vi "Configure Basic Clock Reference.vi"(5 "AES Termination Status (T: Enable)":bool=TRUE, 6 "BNC Termination Status (T: Enable)":bool=TRUE, 7 "Delay Output From Reference (0 s)":dbl, 8 "error in (no error)":errorcluster, 9 "Enable Clock Lock (T: Enable)":bool=TRUE, 10 "Clock Source (0: crAES)":i32(ring) items=["crAES", "crExt", "crInt", "crNTSC", "crSECAM", "crPAL"], 11 "VISA resource name":refnum<visa-resource-name>) -> (0 "error out":errorcluster, 3 "VISA resource name out":refnum<visa-resource-name>)   [LabVIEW 2014, in "Stanford Research SR1.lvlib"]
doc: "Configures the basic attributes for the Clock Reference."
uses:
  Stanford Research SR1.lvlib
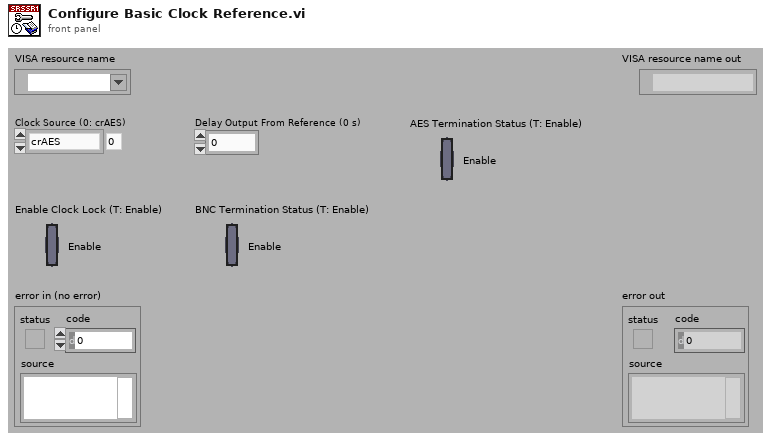
[diagram p1: front panel]
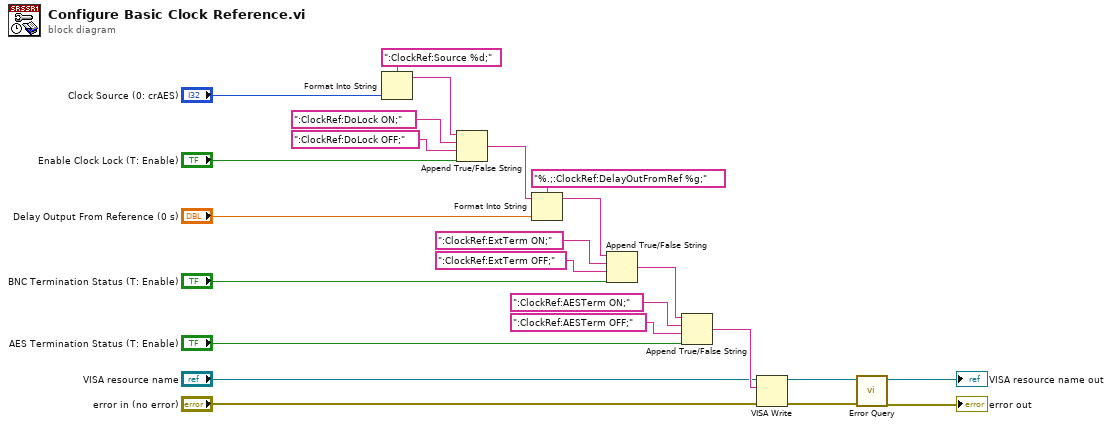
[diagram p0: block diagram]
diagram:
  n1 = Format Into String(format string=":ClockRef:Source %d;", "Clock Source (0: crAES)") -> (resulting string=w22:string)  [unwired: 2 in, 1 out]
  n2 = Append True/False String(1:"Enable Clock Lock (T: Enable)", 2:":ClockRef:DoLock OFF;", 3:":ClockRef:DoLock ON;", 4:w22) -> (0:w18:string)
  n3 = Format Into String(format string="%.;:ClockRef:DelayOutFromRef %g;", initial string=w18, "Delay Output From Reference (0 s)") -> (resulting string=w15:string)  [unwired: 1 in, 1 out]
  n4 = Append True/False String(1:"BNC Termination Status (T: Enable)", 2:":ClockRef:ExtTerm OFF;", 3:":ClockRef:ExtTerm ON;", 4:w15) -> (0:w11:string)
  n5 = Append True/False String(1:"AES Termination Status (T: Enable)", 2:":ClockRef:AESTerm OFF;", 3:":ClockRef:AESTerm ON;", 4:w11) -> (0:w7:string)
  n6 = VISA Write(VISA resource name="VISA resource name", write buffer=w7, error in (no error)="error in (no error)") -> (VISA resource name out=w4:refnum<visa-resource-name>, error out=w3:errorcluster)  [unwired: 1 out]
  n7 = call "Error Query.vi"("error in (no error)"=w3, "VISA resource name"=w4) -> ("error out"=→"error out":errorcluster, "VISA resource name out"=→"VISA resource name out":refnum<visa-resource-name>)  [unwired: 6 in, 2 out]
